vi "FPGAcode.vi"() -> ()   [LabVIEW 2013]
uses:
  <vilib>/Platform/TimedLoop/XDataNode/timing_clust.ctl
  <vilib>/Platform/TimedLoop/XDataNode/nitl_modes.ctl
  <vilib>/Platform/TimedLoop/XDataNode/wakeup.ctl
  <vilib>/rvi/Emulation/niFpgaSctlEmulationGetInTimedLoop.vi
  <vilib>/rvi/Emulation/niFpgaEmulationReportErrorSimple.vi
  <vilib>/rvi/Emulation/niFpgaGetClockAttributes.vi
  <vilib>/rvi/Emulation/niFpgaCriticalErrorInLSC.vi
  <vilib>/rvi/eio/common/nirviEmuTemplateMethod_errors.vi
  <vilib>/Platform/TimedLoop/XDataNode/XDataNode.xnode
  <vilib>/eio/EIONode/EIONode.xnode
  <vilib>/Platform/TimedLoop/XDataNode/XDNodeRunTimeDep.lvlib
panel:
  out "Del Not Armed?":bool
  out "Not Armed?":bool
  in  "Reset One Shot":bool
  in  "One Shot":bool
  out "Filter 1 Detector 3 Correlation":i32
  in  "Filter 2 threshold":i32=1000
  out "Filter 2 Detector 3 Correlation":i32
  in  "Filter 1 threshold":i32=1000
  in  "Filter 3 threshold":i32=1000
  out "Filter 3 Detector 3 Correlation":i32
  in  "Filter 4 threshold":i32=1000
  out "Filter 4 Detector 3 Correlation":i32
  in  "Filter 5 threshold":i32
  out "Filter 5 Detector 3 Correlation":i32
  in  "Filter 6 threshold":i32
  out "Filter 6 Detector 3 Correlation":i32
  in  "Filter 7 threshold":i32
  out "Filter 7 Detector 3 Correlation":i32
  out "Plates":bool
  in  "High Charge Limit":i16
  in  "Low Charge Limit":i16
  in  "High Velocity Count":i32
  in  "Low Velocity Count":i32
  in  "High Mass Limit":i64
  in  "Low Mass Limit":i64
  in  "Mult1":fxp<+,16,7>
  out "Delay1":bool
  out "IO Module\\AI 0":i16
  out "IO Module\\AI 1":i16
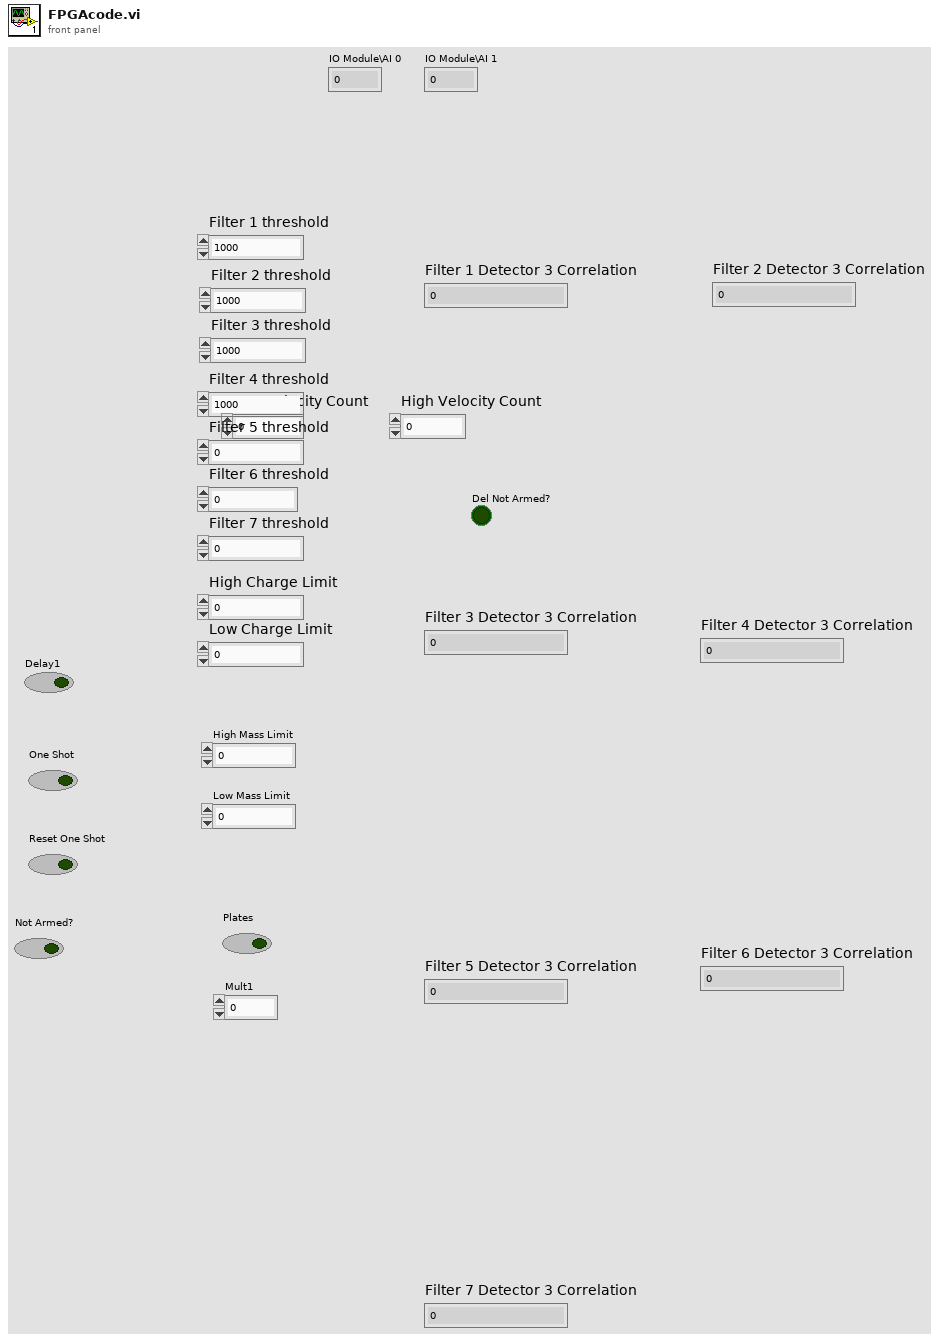
[diagram p1: front panel]
types:
  T1 = typedef "XDNodeRunTimeDep.lvlib/timing_clust.ctl" = cluster{"Expected End [f-1]":u64, "Actual End [f-1]":u64, "Finished Late? [f-1]":bool, "Expected End [i-1]":u64, "Actual End [i-1]":u64, "Finished Late? [i-1]":bool, "Expected Start [i]":u64, "Actual Start [i]":u64, "Expected Start [f]":u64, "Actual Start [f]":u64, "Source Name":string, "Structure Name":string, "Period":i64, "Deadline":i64, "Offset":i64, "Start":i64, "Priority":i32, "Timeout":i32, "Mode":T2, "Wakeup Reason":T3, "Error":errorcluster, "Source Type":string, "Secondary Source Type":string, "Global End Time":u64, "Global Start Time":u64, "Frame Duration":u64, "Iteration Duration":u64, "Assigned CPU":i32, "I/O Scan Engine Mode":u32}
  T2 = typedef "XDNodeRunTimeDep.lvlib/nitl_modes.ctl" = enum32{"No Change", "Process missed periods, maintain original phase", "Discard missed periods, maintain original phase", "Process missed periods, ignore original phase", "Discard missed periods, ignore original phase"}
  T3 = typedef "XDNodeRunTimeDep.lvlib/wakeup.ctl" = enum32{"Normal", "Aborted", "Asynchronous wakeup", "Timing source error", "Timed loop error", "Timeout"}
  T4 = cluster{"Separation cut off 1":i32, "Filter Number":i32, "Separation cut off 2":i32}
  T5 = cluster{"Old Average":i32, "New Average":i32, "Current State":u8, "Detector 1 Correlation":i32, "Detector 3 Correlation":i32, "Velocity Count":i32, "Detector Counter in":i32, "Timeout Count in":i32, "Measured Charge in":i32, "Filter Threshold":i32, "High Correlation in":i32, "Offset":i32, "Offset Average":i32, "Measured Velocity In":i32, "Mult Cluster":cluster{"Mult1":fxp<+,16,7>, "Mult1 Use?":bool}, "Final Delay Count In":u16, "Delay1 In":i32}
  T6 = cluster{"High Charge Limit":i16, "Low Charge Limit":i16, "Low Velocity Count":i32, "High Velocity Count":i32, "Low Velocity Count":i32, fxp<+,30,25>, "High Mass Limit":i64, "Low Mass Limit":i64}
  T7 = cluster{"Average Out":i32, "Next State":u8, "Velocity Count out":i32, "Detector counter out":i32, "Timeout count out":u32, "Measured Charge Out":i32, "High Correlation Out":i32, "Plates":bool, "Offset Out":i32, "Measured Velocity Out":i32, "Final Delay Count Out":u16, "Out1":bool, "Delay1":i32}
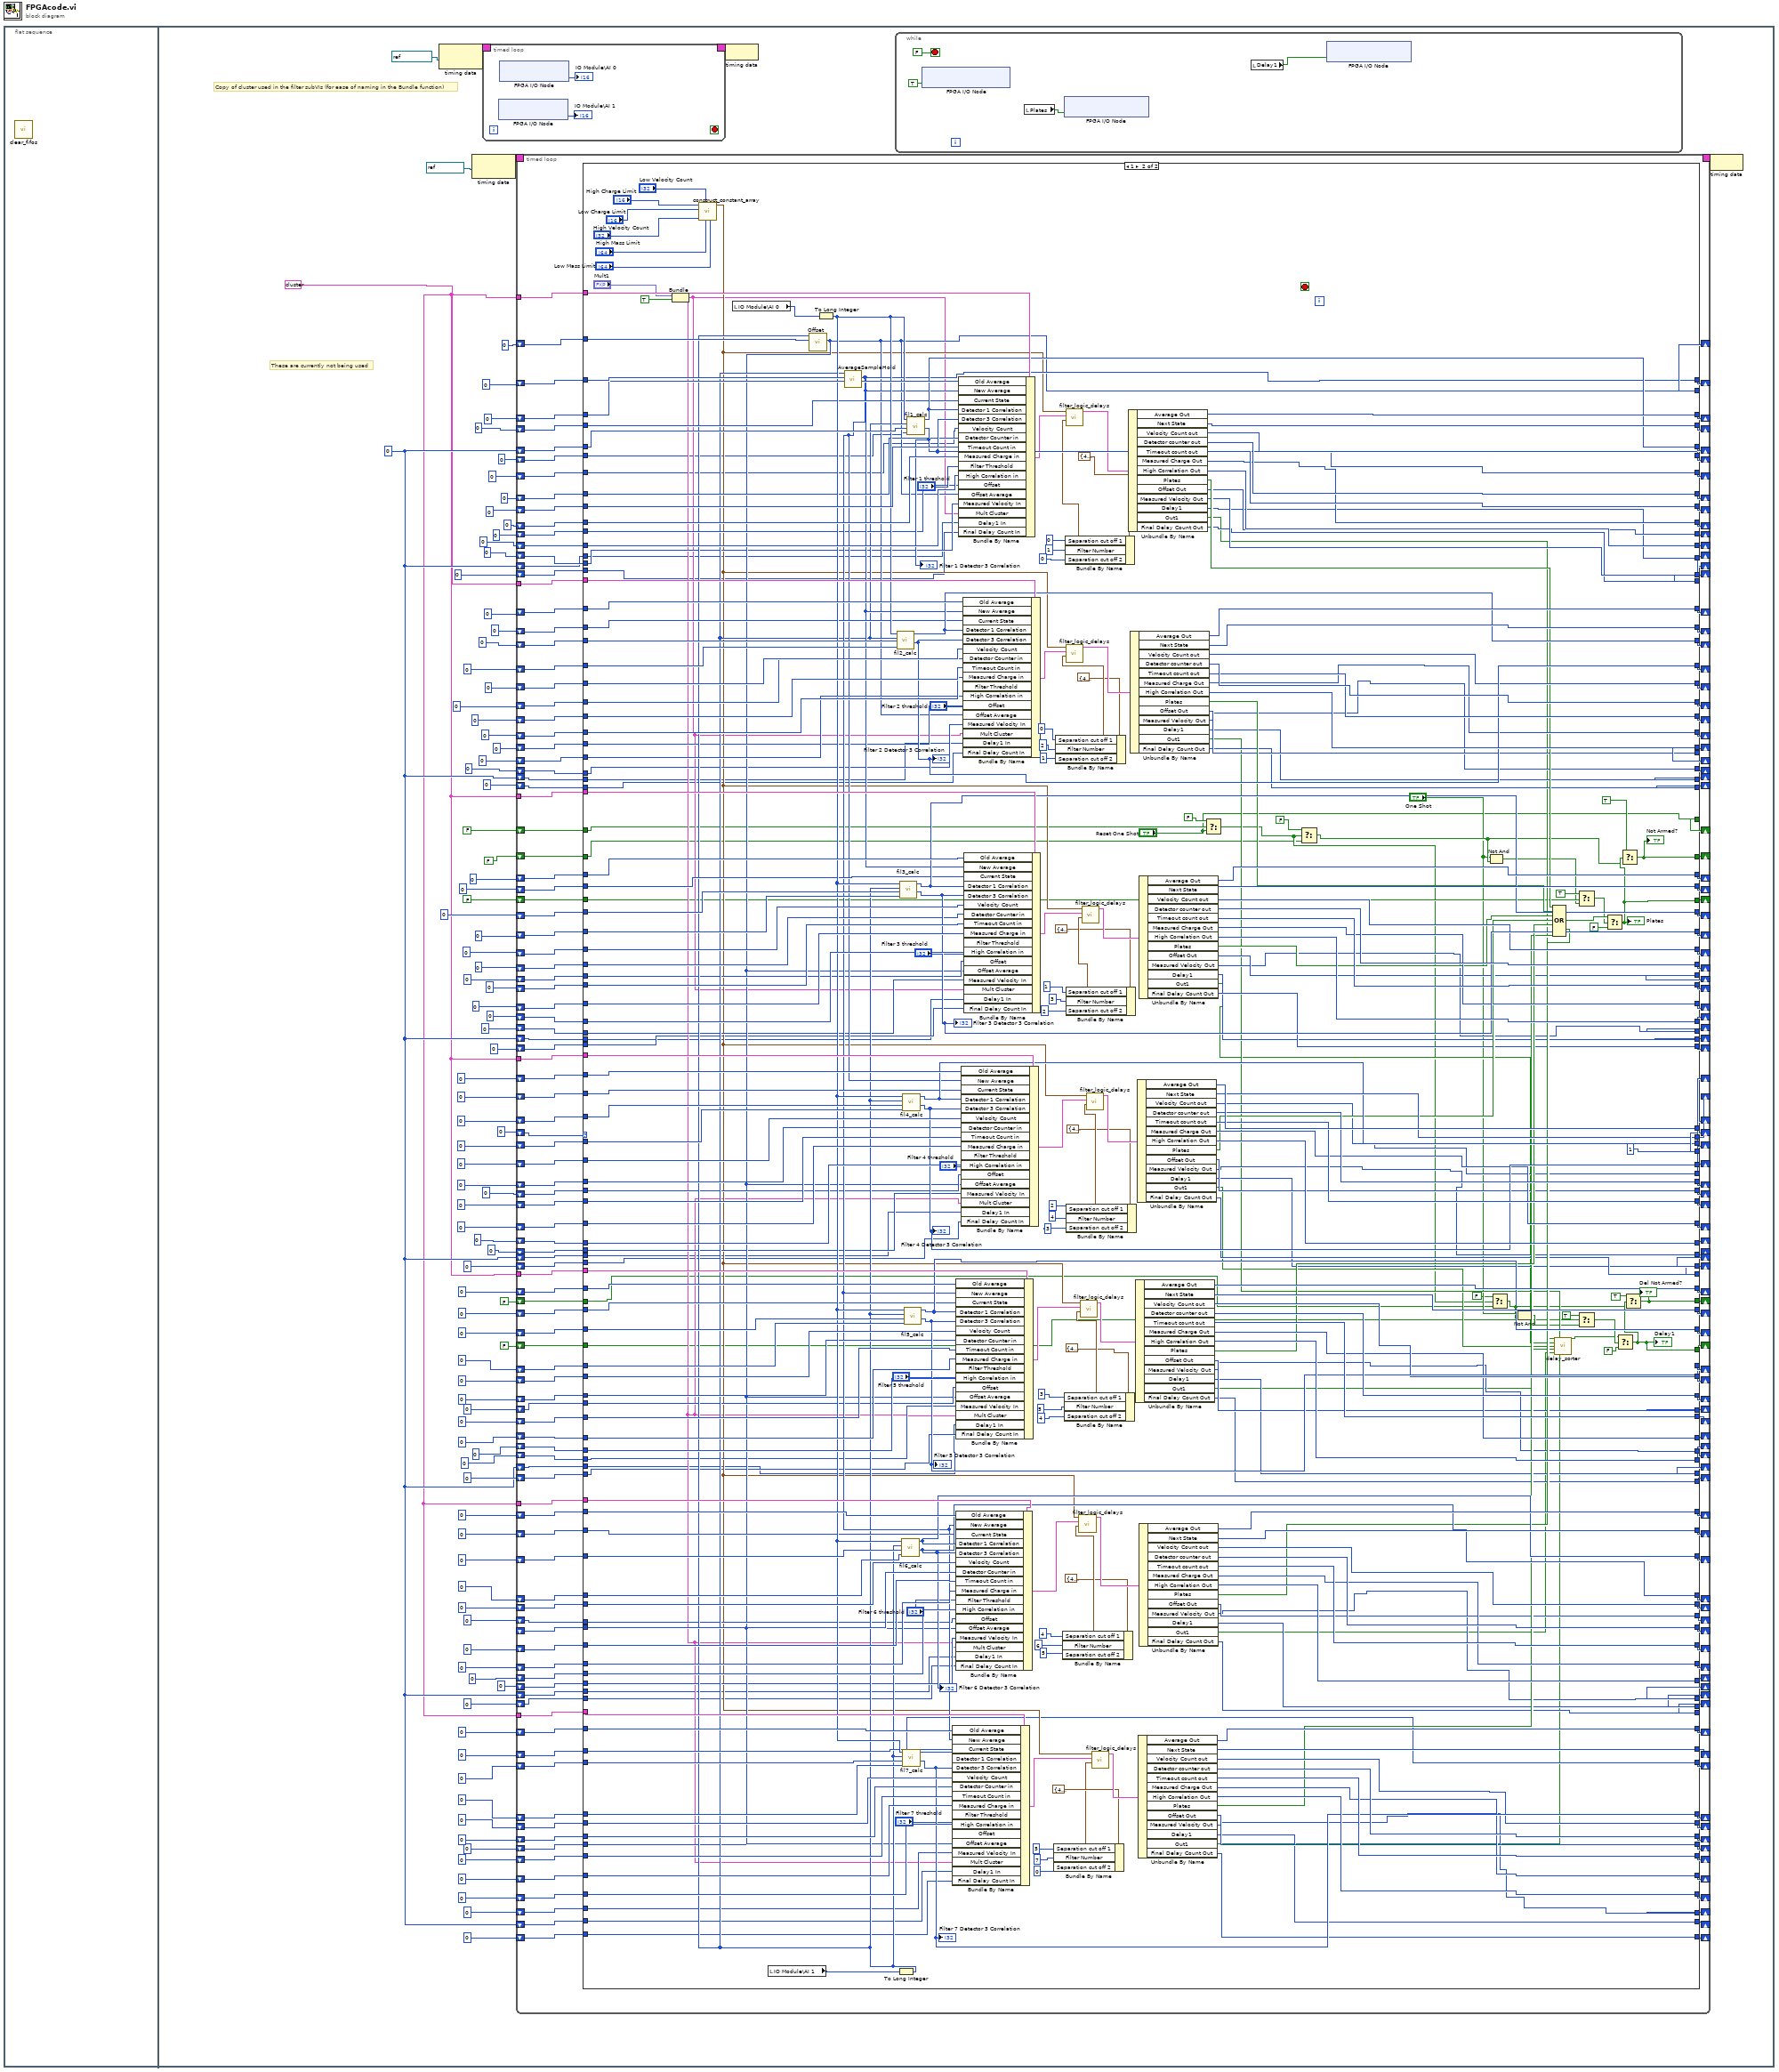
[diagram p0: block diagram]
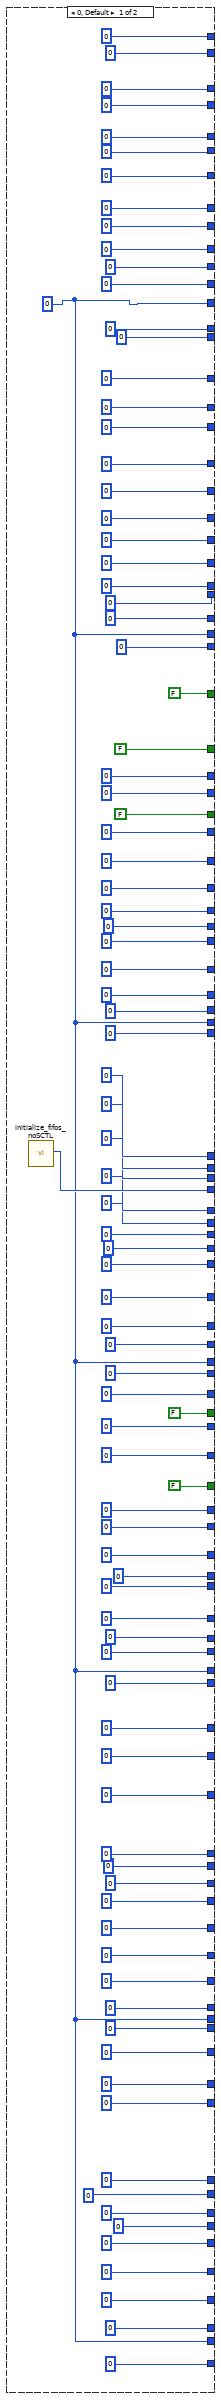
[diagram p2: hidden frame]
diagram:
  n1 = flat-sequence {
    frame #0 {
      n2 = call "clear_fifos.vi"() -> ()  [unwired: 1 in]
    }
    frame #1 {
      w4 = T5 {"Old Average"=0, "New Average"=0, "Current State"=0, "Detector 1 Correlation"=0, "Detector 3 Correlation"=0, "Velocity Count"=0, "Detector Counter in"=0, "Timeout Count in"=0, "Measured Charge in"=0, "Filter Threshold"=0, "High Correlation in"=0, "Offset"=0, "Offset Average"=0, "Measured Velocity In"=0, "Mult Cluster"={"Mult1"=0.0, "Mult1 Use?"=FALSE}, "Final Delay Count In"=0, "Delay1 In"=0} ("Variables Cluster")
      w7 = 0 ("Detector 1 Correlation Out")
      # "These are currently not being used"
      # "Copy of cluster used in the filter subVIs (for ease of naming in the Bundle function)"
      n3 = node-c288(refnum<k21> "AI Clock" ("Source Name")) -> (w34:T1)
      n4 = node-c288(refnum<k21> "26 MHz" ("Source Name")) -> (w98:T1)
      n5 = timed-loop {
        timing: w34 -> [_]
        timing-out: [_] -> w33
        stop <- _ stop-if-true
        n6 = xnode "FPGA I/O Node"() -> ("IO Module\\AI 1"=→"IO Module\\AI 1":i16)  [unwired: 1 in, 1 out]
        n7 = xnode "FPGA I/O Node"() -> ("IO Module\\AI 0"=→"IO Module\\AI 0":i16)  [unwired: 1 in, 1 out]
      }
      n8 = timed-loop {
        timing: w98 -> [_]
        timing-out: [_] -> w97
        shift-right: [w308] -> _
        shift-left: 0 ("Velocity Count out") -> [w230]
        shift-right: [w309] -> _
        shift-left: 0 ("Detector 1 Correlation out") -> [w231]
        shift-right: [w195] -> _
        shift-left: 0 ("Detector counter out") -> [w232]
        shift-right: [w226] -> _
        shift-left: 0 ("Next State") -> [w233]
        shift-right: [w194] -> _
        shift-left: 0 ("Detector 3 Correlation out") -> [w229]
        shift-right: [w307] -> _
        shift-left: 0 ("Timeout count out") -> [w228]
        shift-right: [w222] -> _
        shift-left: 0 ("Next State") -> [w225]
        shift-right: [w221] -> _
        shift-left: 0 ("Detector counter out") -> [w224]
        shift-right: [w193] -> _
        shift-left: 0 ("Detector 1 Correlation out") -> [w301]
        shift-right: [w298] -> _
        shift-left: 0 ("Velocity Count out") -> [w300]
        shift-right: [w297] -> _
        shift-left: u32 0 ("Detector 3 Correlation out") -> [w299]
        shift-right: [w292] -> _
        shift-left: 0 ("Timeout count out") -> [w293]
        shift-right: [w216] -> _
        shift-left: 0 ("Next State") -> [w219]
        shift-right: [w191] -> _
        shift-left: 0 ("Detector counter out") -> [w289]
        shift-right: [w287] -> _
        shift-left: 0 ("Detector 1 Correlation out") -> [w288]
        shift-right: [w285] -> _
        shift-left: u32 0 ("Velocity Count out") -> [w286]
        shift-right: [w190] -> _
        shift-left: 0 ("Detector 3 Correlation out") -> [w284]
        shift-right: [w283] -> _
        shift-left: 0 ("Timeout count out") -> [w218]
        shift-right: [w310] -> _
        shift-left: u8 0 ("High Correlation Out") -> [w313]
        shift-right: [w302] -> _
        shift-left: u8 0 ("High Correlation Out") -> [w303]
        shift-right: [w217] -> _
        shift-left: 0 ("High Correlation Out") -> [w220]
        shift-right: [w311] -> _
        shift-left: 0 ("Measured Charge Out") -> [w314]
        shift-right: [w304] -> _
        shift-left: 0 ("Measured Charge Out") -> [w305]
        shift-right: [w291] -> _
        shift-left: u8 0 ("Measured Charge Out") -> [w290]
        shift-right: [w181] -> _
        shift-left: 0 ("Output New Average") -> [w315]
        shift-right: [w227] -> _
        shift-left: w7 -> [w234]
        tunnel: w4 -> [w312]
        shift-right: [w192] -> _
        shift-left: 0 ("High Sample Out") -> [w295]
        shift-right: [w296] -> _
        shift-left: 0 ("High Correlation Out") -> [w223]
        tunnel: w4 -> [w306]
        tunnel: w4 -> [w294]
        shift-right: [w282] -> _
        shift-left: 0 ("Average Out") -> [w281]
        shift-right: [w280] -> _
        shift-left: u8 0 ("Next State") -> [w279]
        shift-right: [w212] -> _
        shift-left: 0 ("Detector 1 Correlation out") -> [w214]
        shift-right: [w211] -> _
        shift-left: 0 ("Detector 3 Correlation out") -> [w213]
        shift-right: [w189] -> _
        shift-left: 0 ("Velocity Count out") -> [w278]
        shift-right: [w277] -> _
        shift-left: 0 ("Detector counter out") -> [w276]
        shift-right: [w275] -> _
        shift-left: u32 0 ("Timeout count out") -> [w274]
        shift-right: [w188] -> _
        shift-left: 0 ("Measured Charge Out") -> [w273]
        shift-right: [w272] -> _
        shift-left: 0 ("High Correlation Out") -> [w215]
        tunnel: w4 -> [w271]
        shift-right: [w269] -> _
        shift-left: 0 ("Average Out") -> [w268]
        shift-right: [w267] -> _
        shift-left: u8 0 ("Next State") -> [w266]
        shift-right: [w207] -> _
        shift-left: 0 ("Detector 1 Correlation out") -> [w210]
        shift-right: [w206] -> _
        shift-left: 0 ("Detector 3 Correlation out") -> [w209]
        shift-right: [w187] -> _
        shift-left: 0 ("Velocity Count out") -> [w265]
        shift-right: [w264] -> _
        shift-left: 0 ("Detector counter out") -> [w263]
        shift-right: [w262] -> _
        shift-left: u32 0 ("Timeout count out") -> [w261]
        shift-right: [w186] -> _
        shift-left: 0 ("Measured Charge Out") -> [w260]
        shift-right: [w259] -> _
        shift-left: 0 ("High Correlation Out") -> [w208]
        tunnel: w4 -> [w270]
        shift-right: [w257] -> _
        shift-left: 0 ("Average Out") -> [w255]
        shift-right: [w256] -> _
        shift-left: u8 0 ("Next State") -> [w252]
        shift-right: [w202] -> _
        shift-left: 0 ("Detector 1 Correlation out") -> [w205]
        shift-right: [w201] -> _
        shift-left: 0 ("Detector 3 Correlation out") -> [w204]
        shift-right: [w184] -> _
        shift-left: 0 ("Velocity Count out") -> [w254]
        shift-right: [w251] -> _
        shift-left: _ -> [w253]
        shift-right: [w250] -> _
        shift-left: u32 0 ("Timeout count out") -> [w249]
        shift-right: [w185] -> _
        shift-left: 0 ("Measured Charge Out") -> [w248]
        shift-right: [w247] -> _
        shift-left: 0 ("High Correlation Out") -> [w203]
        tunnel: w4 -> [w258]
        shift-right: [w245] -> _
        shift-left: 0 ("Average Out") -> [w244]
        shift-right: [w243] -> _
        shift-left: u8 0 ("Next State") -> [w235]
        shift-right: [w197] -> _
        shift-left: 0 ("Detector 1 Correlation out") -> [w200]
        shift-right: [w196] -> _
        shift-left: 0 ("Detector 3 Correlation out") -> [w199]
        shift-right: [w183] -> _
        shift-left: 0 ("Velocity Count out") -> [w242]
        shift-right: [w241] -> _
        shift-left: 0 ("Detector counter out") -> [w240]
        shift-right: [w239] -> _
        shift-left: u32 0 ("Timeout count out") -> [w238]
        shift-right: [w182] -> _
        shift-left: 0 ("Measured Charge Out") -> [w237]
        shift-right: [w236] -> _
        shift-left: 0 ("High Correlation Out") -> [w198]
        tunnel: w4 -> [w246]
        shift-right: [w179] -> _
        shift-left: i16 0 -> [w180]
        shift-right: [w177] -> _
        shift-left: 0 -> [w178]
        shift-right: [w176] -> _
        shift-left: 0 -> [w173]
        shift-right: [w174] -> _
        shift-left: 0 -> [w175]
        shift-right: [w171] -> _
        shift-left: 0 ("Offset Out") -> [w172]
        shift-right: [w170] -> _
        shift-left: 0 ("Offset Out") -> [w169]
        shift-right: [w168] -> _
        shift-left: 0 ("Offset Out") -> [w167]
        shift-right: [w166] -> _
        shift-left: 0 ("Offset Out") -> [w165]
        shift-right: [w164] -> _
        shift-left: 0 ("Offset Out") -> [w163]
        shift-right: [w161] -> _
        shift-left: 0 -> [w162]
        shift-right: [w160] -> _
        shift-left: 0 -> [w149]
        shift-right: [w159] -> _
        shift-left: 0 -> [w150]
        shift-right: [w158] -> _
        shift-left: 0 -> [w151]
        shift-right: [w157] -> _
        shift-left: 0 -> [w152]
        shift-right: [w156] -> _
        shift-left: 0 -> [w153]
        shift-right: [w155] -> _
        shift-left: 0 ("Measured Velocity Out") -> [w154]
        shift-right: [w148] -> _
        shift-left: w7 -> [w146]
        shift-right: [w147] -> _
        shift-left: u32 0 ("Final Delay Count Out") -> [w145]
        shift-right: [w144] -> _
        shift-left: w7 -> [w142]
        shift-right: [w143] -> _
        shift-left: u32 0 ("Final Delay Count Out") -> [w141]
        shift-right: [w140] -> _
        shift-left: w7 -> [w138]
        shift-right: [w139] -> _
        shift-left: u32 0 ("Final Delay Count Out") -> [w137]
        shift-right: [w136] -> _
        shift-left: w7 -> [w134]
        shift-right: [w135] -> _
        shift-left: u32 0 ("Final Delay Count Out") -> [w133]
        shift-right: [w132] -> _
        shift-left: w7 -> [w130]
        shift-right: [w131] -> _
        shift-left: u32 0 ("Final Delay Count Out") -> [w129]
        shift-right: [w128] -> _
        shift-left: w7 -> [w126]
        shift-right: [w127] -> _
        shift-left: u32 0 ("Final Delay Count Out") -> [w125]
        shift-right: [w124] -> _
        shift-left: w7 -> [w122]
        shift-right: [w123] -> _
        shift-left: u32 0 ("Final Delay Count Out") -> [w121]
        shift-right: [w119] -> _
        shift-left: FALSE -> [w120]
        shift-right: [w118] -> _
        shift-left: FALSE ("f") -> [w117]
        shift-right: [w116] -> _
        shift-left: FALSE ("Reset One Shot") -> [w115]
        shift-right: [w111] -> _
        shift-left: FALSE -> [w114]
        shift-right: [w112] -> _
        shift-left: FALSE -> [w113]
        stop <- _ stop-if-true
        n9 = case shown="1" w180 {
          tunnel: w315 -> [_ w715]
          tunnel: w314 -> [_ w714]
          tunnel: w313 -> [_ w549]
          tunnel: w312 -> [_ w713]
          tunnel: [0 ("Average Out") w712] -> w311
          tunnel: [u16 0 ("Next State") w711] -> w310
          tunnel: [0 ("Detector counter out") w710] -> w309
          tunnel: [u32 0 ("Timeout count out") w709] -> w308
          tunnel: [0 ("High Correlation Out") w708] -> w307
          tunnel: w306 -> [_ w707]
          tunnel: w305 -> [_ w706]
          tunnel: [0 ("Average Out") w705] -> w304
          tunnel: w303 -> [_ w548]
          tunnel: [u16 0 ("Next State") w704] -> w302
          tunnel: w301 -> [_ w703]
          tunnel: w300 -> [_ w541]
          tunnel: w299 -> [_ w702]
          tunnel: [0 ("Detector counter out") w701] -> w298
          tunnel: [u32 0 ("Timeout count out") w700] -> w297
          tunnel: [0 ("High Correlation Out") w699] -> w296
          tunnel: w295 -> [_ w698]
          tunnel: w294 -> [_ w697]
          tunnel: w293 -> [_ w696]
          tunnel: [0 ("Average Out") w695] -> w292
          tunnel: [u16 0 ("Next State") w694] -> w291
          tunnel: w290 -> [_ w547]
          tunnel: w289 -> [_ w693]
          tunnel: w288 -> [_ w540]
          tunnel: [0 ("Detector counter out") w692] -> w287
          tunnel: w286 -> [_ w691]
          tunnel: [u32 0 ("Timeout count out") w690] -> w285
          tunnel: w284 -> [_ w689]
          tunnel: [0 ("High Correlation Out") w688] -> w283
          tunnel: [0 ("Average Out") w687] -> w282
          tunnel: w281 -> [_ w686]
          tunnel: [u16 0 ("Next State") w685] -> w280
          tunnel: w279 -> [_ w546]
          tunnel: w278 -> [_ w684]
          tunnel: [0 ("Detector counter out") w683] -> w277
          tunnel: w276 -> [_ w539]
          tunnel: [u32 0 ("Timeout count out") w682] -> w275
          tunnel: w274 -> [_ w681]
          tunnel: w273 -> [_ w680]
          tunnel: [0 ("High Correlation Out") w679] -> w272
          tunnel: w271 -> [_ w678]
          tunnel: w270 -> [_ w677]
          tunnel: [0 ("Average Out") w676] -> w269
          tunnel: w268 -> [_ w675]
          tunnel: [u16 0 ("Next State") w674] -> w267
          tunnel: w266 -> [_ w545]
          tunnel: w265 -> [_ w673]
          tunnel: [0 ("Detector counter out") w672] -> w264
          tunnel: w263 -> [_ w538]
          tunnel: [u32 0 ("Timeout count out") w671] -> w262
          tunnel: w261 -> [_ w670]
          tunnel: w260 -> [_ w669]
          tunnel: [0 ("High Correlation Out") w668] -> w259
          tunnel: w258 -> [_ w667]
          tunnel: [0 ("Average Out") w666] -> w257
          tunnel: [u16 0 ("Next State") w665] -> w256
          tunnel: w255 -> [_ w664]
          tunnel: w254 -> [_ w663]
          tunnel: w253 -> [_ w537]
          tunnel: w252 -> [_ w544]
          tunnel: [0 ("Detector counter out") w662] -> w251
          tunnel: [u32 0 ("Timeout count out") w661] -> w250
          tunnel: w249 -> [_ w660]
          tunnel: w248 -> [_ w659]
          tunnel: [0 ("High Correlation Out") w658] -> w247
          tunnel: w246 -> [_ w657]
          tunnel: [0 ("Average Out") w656] -> w245
          tunnel: w244 -> [_ w655]
          tunnel: [u16 0 ("Next State") w654] -> w243
          tunnel: w242 -> [_ w653]
          tunnel: [0 ("Detector counter out") w652] -> w241
          tunnel: w240 -> [_ w536]
          tunnel: [u32 0 ("Timeout count out") w651] -> w239
          tunnel: w238 -> [_ w650]
          tunnel: w237 -> [_ w649]
          tunnel: [0 ("High Correlation Out") w648] -> w236
          tunnel: w235 -> [_ w543]
          tunnel: w234 -> [_ w647]
          tunnel: w233 -> [_ w444]
          tunnel: w232 -> [_ w445]
          tunnel: w231 -> [_ w542]
          tunnel: w230 -> [_ w646]
          tunnel: w229 -> [_ w645]
          tunnel: w228 -> [_ w644]
          tunnel: [0 ("Detector 1 Correlation Out") w643] -> w227
          tunnel: [0 ("Detector 3 Correlation Out") w642] -> w226
          tunnel: w225 -> [_ w641]
          tunnel: w224 -> [_ w640]
          tunnel: w223 -> [_ w639]
          tunnel: [0 ("Detector 1 Correlation Out") w638] -> w222
          tunnel: [0 ("Detector 3 Correlation Out") w637] -> w221
          tunnel: w220 -> [_ w636]
          tunnel: w219 -> [_ w635]
          tunnel: w218 -> [_ w634]
          tunnel: [0 ("Detector 1 Correlation Out") w633] -> w217
          tunnel: [0 ("Detector 3 Correlation Out") w632] -> w216
          tunnel: w215 -> [_ w631]
          tunnel: w214 -> [_ w630]
          tunnel: w213 -> [_ w629]
          tunnel: [0 ("Detector 1 Correlation Out") w628] -> w212
          tunnel: [0 ("Detector 3 Correlation Out") w627] -> w211
          tunnel: w210 -> [_ w626]
          tunnel: w209 -> [_ w625]
          tunnel: w208 -> [_ w624]
          tunnel: [0 ("Detector 1 Correlation Out") w623] -> w207
          tunnel: [0 ("Detector 3 Correlation Out") w622] -> w206
          tunnel: w205 -> [_ w621]
          tunnel: w204 -> [_ w620]
          tunnel: w203 -> [_ w619]
          tunnel: [0 ("Detector 1 Correlation Out") w618] -> w202
          tunnel: [0 ("Detector 3 Correlation Out") w617] -> w201
          tunnel: w200 -> [_ w616]
          tunnel: w199 -> [_ w615]
          tunnel: w198 -> [_ w614]
          tunnel: [0 ("Detector 1 Correlation Out") w479] -> w197
          tunnel: [0 ("Detector 3 Correlation Out") w613] -> w196
          tunnel: [0 ("Velocity Count out") w612] -> w195
          tunnel: [0 ("Measured Charge Out") w611] -> w194
          tunnel: [0 ("Velocity Count out") w610] -> w193
          tunnel: [0 ("Measured Charge Out") w609] -> w192
          tunnel: [0 ("Velocity Count out") w608] -> w191
          tunnel: [0 ("Measured Charge Out") w607] -> w190
          tunnel: [0 ("Velocity Count out") w535] -> w189
          tunnel: [0 ("Measured Charge Out") w606] -> w188
          tunnel: [0 ("Velocity Count out") w605] -> w187
          tunnel: [0 ("Measured Charge Out") w604] -> w186
          tunnel: [0 ("Measured Charge Out") w603] -> w185
          tunnel: [0 ("Velocity Count out") w602] -> w184
          tunnel: [0 ("Velocity Count out") w601] -> w183
          tunnel: [0 ("Measured Charge Out") w600] -> w182
          tunnel: [0 ("Output New Average") w534] -> w181
          tunnel: [w408 i16 1 ("Output State")] -> w179
          tunnel: w178 -> [_ w531]
          tunnel: [0 ("Offset Out") w530] -> w177
          tunnel: [0 ("Offset Out") w529] -> w176
          tunnel: w175 -> [_ w528]
          tunnel: [0 ("Output New Average") w517] -> w174
          tunnel: w173 -> [_ w526]
          tunnel: w172 -> [_ w525]
          tunnel: [0 ("Offset Out") w524] -> w171
          tunnel: [0 ("Offset Out") w523] -> w170
          tunnel: w169 -> [_ w522]
          tunnel: [0 ("Offset Out") w521] -> w168
          tunnel: w167 -> [_ w520]
          tunnel: [0 ("Offset Out") w519] -> w166
          tunnel: w165 -> [_ w518]
          tunnel: [0 ("Offset Out") w516] -> w164
          tunnel: w163 -> [_ w515]
          tunnel: w162 -> [_ w510]
          tunnel: [0 ("Measured Velocity Out") w503] -> w161
          tunnel: [0 ("Measured Velocity Out") w502] -> w160
          tunnel: [0 ("Measured Velocity Out") w501] -> w159
          tunnel: [0 ("Measured Velocity Out") w500] -> w158
          tunnel: [0 ("Measured Velocity Out") w499] -> w157
          tunnel: [0 ("Measured Velocity Out") w498] -> w156
          tunnel: [0 ("Measured Velocity Out") w497] -> w155
          tunnel: w154 -> [_ w509]
          tunnel: w153 -> [_ w508]
          tunnel: w152 -> [_ w507]
          tunnel: w151 -> [_ w506]
          tunnel: w150 -> [_ w505]
          tunnel: w149 -> [_ w504]
          tunnel: [w321 w474] -> w148
          tunnel: [u32 0 ("Final Delay Count Out") w492] -> w147
          tunnel: w146 -> [_ w491]
          tunnel: w145 -> [_ w490]
          tunnel: [w321 w489] -> w144
          tunnel: [u32 0 ("Final Delay Count Out") w488] -> w143
          tunnel: w142 -> [_ w487]
          tunnel: w141 -> [_ w486]
          tunnel: [w321 w473] -> w140
          tunnel: [u32 0 ("Final Delay Count Out") w485] -> w139
          tunnel: w138 -> [_ w466]
          tunnel: w137 -> [_ w484]
          tunnel: [w321 w472] -> w136
          tunnel: [u32 0 ("Final Delay Count Out") w483] -> w135
          tunnel: w134 -> [_ w465]
          tunnel: w133 -> [_ w482]
          tunnel: [w321 w471] -> w132
          tunnel: [u32 0 ("Final Delay Count Out") w481] -> w131
          tunnel: w130 -> [_ w464]
          tunnel: w129 -> [_ w480]
          tunnel: [w321 w470] -> w128
          tunnel: [u32 0 ("Final Delay Count Out") w478] -> w127
          tunnel: w126 -> [_ w463]
          tunnel: w125 -> [_ w477]
          tunnel: [w321 w469] -> w124
          tunnel: [u32 0 ("Final Delay Count Out") w476] -> w123
          tunnel: w122 -> [_ w462]
          tunnel: w121 -> [_ w475]
          tunnel: w120 -> [_ w410]
          tunnel: [FALSE ("t") w430] -> w119
          tunnel: [FALSE ("f") w442] -> w118
          tunnel: w117 -> [_ w441]
          tunnel: [FALSE ("Reset One Shot") "Reset One Shot"] -> w116
          tunnel: w115 -> [_ w428]
          tunnel: w114 -> [_ w411]
          tunnel: w113 -> [_ w417]
          tunnel: [FALSE ("Delay1") w416] -> w112
          tunnel: [FALSE w413] -> w111
          frame 0, Default {
            w321 = 0
            n10 = call "initialize_fifos_noSCTL.vi"() -> ("Output State"=w408:i16)  [unwired: 11 in]
          }
          frame 1 {
            n11 = Bundle("Mult1"="Mult1", TRUE) -> (w493:cluster{"Mult1":fxp<+,16,7>, bool})  [unwired: 1 in]
            n12 = call "construct_constant_array.vi"("Low Mass Limit"="Low Mass Limit", "High Mass Limit"="High Mass Limit", "Low Velocity Count"="Low Velocity Count", "High Velocity Count"="High Velocity Count", "Low Charge Limit"="Low Charge Limit", "High Charge Limit"="High Charge Limit") -> ("constants cluster"=w494:T6)  [unwired: 5 in]
            n13 = local read "IO Module\\AI 0"() -> (w533:i16)
            n14 = local read "IO Module\\AI 1"() -> (w532:i16)
            n15 = To Long Integer(number=w533) -> (32bit integer=w558:i32)
            n16 = To Long Integer(number=w532) -> (32bit integer=w527:i32)
            n17 = call "Offset.vi"("Previous Average"=w528, "Input Value"=w527) -> ("Output New Average"=w517:i32)  [unwired: 7 in]
            n18 = call "AverageSampleHold.vi"("Previous Average"=w715, "Input Value"=w527) -> ("Output New Average"=w534:i32)  [unwired: 7 in]
            n19 = call "fil2_calc.vi"("Detector 3 Correlation In"=w640, "Detector 1 Correlation In"=w641, "AI1"=w527, "AI0"=w558) -> ("Detector 3 Correlation Out"=w637:i32, "Detector 1 Correlation Out"=w638:i32)  [unwired: 4 in]
            "Filter 2 Detector 3 Correlation" <- w637
            n20 = call "fil3_calc.vi"("Detector 3 Correlation In"=w635, "Detector 1 Correlation In"=w636, "AI1"=w527, "AI0"=w558) -> ("Detector 3 Correlation Out"=w632:i32, "Detector 1 Correlation Out"=w633:i32)  [unwired: 4 in]
            "Filter 3 Detector 3 Correlation" <- w632
            n21 = call "fil6_calc.vi"("Detector 3 Correlation In"=w620, "Detector 1 Correlation In"=w621, "AI1"=w527, "AI0"=w558) -> ("Detector 3 Correlation Out"=w617:i32, "Detector 1 Correlation Out"=w618:i32)  [unwired: 4 in]
            "Filter 6 Detector 3 Correlation" <- w617
            n22 = call "fil4_calc.vi"("Detector 3 Correlation In"=w629, "Detector 1 Correlation In"=w630, "AI1"=w527, "AI0"=w558) -> ("Detector 3 Correlation Out"=w627:i32, "Detector 1 Correlation Out"=w628:i32)  [unwired: 4 in]
            "Filter 4 Detector 3 Correlation" <- w627
            n23 = call "fil7_calc.vi"("Detector 3 Correlation In"=w615, "Detector 1 Correlation In"=w616, "AI1"=w527, "AI0"=w558) -> ("Detector 3 Correlation Out"=w613:i32, "Detector 1 Correlation Out"=w479:i32)  [unwired: 4 in]
            "Filter 7 Detector 3 Correlation" <- w613
            n24 = call "fil5_calc.vi"("Detector 3 Correlation In"=w625, "Detector 1 Correlation In"=w626, "AI1"=w527, "AI0"=w558) -> ("Detector 3 Correlation Out"=w622:i32, "Detector 1 Correlation Out"=w623:i32)  [unwired: 4 in]
            "Filter 5 Detector 3 Correlation" <- w622
            n25 = call "fil1_calc.vi"("Detector 3 Correlation In"=w444, "Detector 1 Correlation In"=w647, "AI1"=w527, "AI0"=w558) -> ("Detector 3 Correlation Out"=w642:i32, "Detector 1 Correlation Out"=w643:i32)  [unwired: 4 in]
            "Filter 1 Detector 3 Correlation" <- w642
            n26 = Bundle By Name(cluster=w657, "Old Average"=w655, "New Average"=w534, "Current State"=w543, "Detector 1 Correlation"=w479, "Detector 3 Correlation"=w613, "Velocity Count"=w653, "Detector Counter in"=w536, "Timeout Count in"=w650, "Measured Charge in"=w649, "Filter Threshold"="Filter 7 threshold", "High Correlation in"=w614, "Offset"=w515, "Offset Average"=w517, "Measured Velocity In"=w509, "Mult Cluster"=w493, "Delay1 In"=w462, "Final Delay Count In"=w475) -> (w432:T5)
            n27 = Bundle By Name(cluster=w667, "Old Average"=w664, "New Average"=w534, "Current State"=w544, "Detector 1 Correlation"=w618, "Detector 3 Correlation"=w617, "Velocity Count"=w663, "Detector Counter in"=w537, "Timeout Count in"=w660, "Measured Charge in"=w659, "Filter Threshold"="Filter 6 threshold", "High Correlation in"=w619, "Offset"=w518, "Offset Average"=w517, "Measured Velocity In"=w508, "Mult Cluster"=w493, "Delay1 In"=w463, "Final Delay Count In"=w477) -> (w433:T5)
            n28 = Bundle By Name(cluster=w677, "Old Average"=w675, "New Average"=w534, "Current State"=w545, "Detector 1 Correlation"=w623, "Detector 3 Correlation"=w622, "Velocity Count"=w673, "Detector Counter in"=w538, "Timeout Count in"=w670, "Measured Charge in"=w669, "Filter Threshold"="Filter 5 threshold", "High Correlation in"=w624, "Offset"=w520, "Offset Average"=w517, "Measured Velocity In"=w507, "Mult Cluster"=w493, "Delay1 In"=w464, "Final Delay Count In"=w480) -> (w434:T5)
            n29 = Bundle By Name(cluster=w713, "Old Average"=w714, "New Average"=w534, "Current State"=w549, "Detector 1 Correlation"=w643, "Detector 3 Correlation"=w642, "Velocity Count"=w445, "Detector Counter in"=w542, "Timeout Count in"=w646, "Measured Charge in"=w645, "Filter Threshold"="Filter 1 threshold", "High Correlation in"=w644, "Offset"=w531, "Offset Average"=w517, "Measured Velocity In"=w510, "Mult Cluster"=w493, "Delay1 In"=w491, "Final Delay Count In"=w490) -> (w438:T5)
            n30 = Bundle By Name(cluster=w678, "Old Average"=w686, "New Average"=w534, "Current State"=w546, "Detector 1 Correlation"=w628, "Detector 3 Correlation"=w627, "Velocity Count"=w684, "Detector Counter in"=w539, "Timeout Count in"=w681, "Measured Charge in"=w680, "Filter Threshold"="Filter 4 threshold", "High Correlation in"=w631, "Offset"=w522, "Offset Average"=w517, "Measured Velocity In"=w506, "Mult Cluster"=w493, "Delay1 In"=w465, "Final Delay Count In"=w482) -> (w435:T5)
            n31 = Bundle By Name(cluster=w707, "Old Average"=w706, "New Average"=w534, "Current State"=w548, "Detector 1 Correlation"=w638, "Detector 3 Correlation"=w637, "Velocity Count"=w703, "Detector Counter in"=w541, "Timeout Count in"=w702, "Measured Charge in"=w698, "Filter Threshold"="Filter 2 threshold", "High Correlation in"=w639, "Offset"=w526, "Offset Average"=w517, "Measured Velocity In"=w504, "Mult Cluster"=w493, "Delay1 In"=w487, "Final Delay Count In"=w486) -> (w437:T5)
            n32 = Bundle By Name(cluster=w697, "Old Average"=w696, "New Average"=w534, "Current State"=w547, "Detector 1 Correlation"=w633, "Detector 3 Correlation"=w632, "Velocity Count"=w693, "Detector Counter in"=w540, "Timeout Count in"=w691, "Measured Charge in"=w689, "Filter Threshold"="Filter 3 threshold", "High Correlation in"=w634, "Offset"=w525, "Offset Average"=w517, "Measured Velocity In"=w505, "Mult Cluster"=w493, "Delay1 In"=w466, "Final Delay Count In"=w484) -> (w436:T5)
            n33 = Bundle By Name(cluster=T4 {"Separation cut off 1"=4, "Filter Number"=5, "Separation cut off 2"=6} ("Filter Specific Constants"), "Separation cut off 1"=5, "Filter Number"=7, "Separation cut off 2"=0) -> (w448:T4)
            n34 = Bundle By Name(cluster=T4 {"Separation cut off 1"=4, "Filter Number"=5, "Separation cut off 2"=6} ("Filter Specific Constants"), "Separation cut off 1"=0, "Filter Number"=2, "Separation cut off 2"=1) -> (w591:T4)
            n35 = Bundle By Name(cluster=T4 {"Separation cut off 1"=4, "Filter Number"=5, "Separation cut off 2"=6} ("Filter Specific Constants"), "Separation cut off 1"=4, "Filter Number"=6, "Separation cut off 2"=5) -> (w581:T4)
            n36 = Bundle By Name(cluster=T4 {"Separation cut off 1"=4, "Filter Number"=5, "Separation cut off 2"=6} ("Filter Specific Constants"), "Separation cut off 1"=3, "Filter Number"=5, "Separation cut off 2"=4) -> (w583:T4)
            n37 = Bundle By Name(cluster=T4 {"Separation cut off 1"=4, "Filter Number"=5, "Separation cut off 2"=6} ("Filter Specific Constants"), "Separation cut off 1"=0, "Filter Number"=1, "Separation cut off 2"=0) -> (w589:T4)
            n38 = call "filter_logic_delays.vi"("Filter Specific Constants"=w589, "Variables Cluster"=w438, "controls cluster"=w494) -> ("Output Cluster"=w588:T7)  [unwired: 8 in]
            n39 = call "filter_logic_delays.vi"("Filter Specific Constants"=w591, "Variables Cluster"=w437, "controls cluster"=w494) -> ("Output Cluster"=w598:T7)  [unwired: 8 in]
            n40 = Bundle By Name(cluster=T4 {"Separation cut off 1"=4, "Filter Number"=5, "Separation cut off 2"=6} ("Filter Specific Constants"), "Separation cut off 1"=1, "Filter Number"=3, "Separation cut off 2"=2) -> (w587:T4)
            n41 = Bundle By Name(cluster=T4 {"Separation cut off 1"=4, "Filter Number"=5, "Separation cut off 2"=6} ("Filter Specific Constants"), "Separation cut off 1"=2, "Filter Number"=4, "Separation cut off 2"=3) -> (w585:T4)
            n42 = call "filter_logic_delays.vi"("Filter Specific Constants"=w581, "Variables Cluster"=w433, "controls cluster"=w494) -> ("Output Cluster"=w580:T7)  [unwired: 8 in]
            n43 = call "filter_logic_delays.vi"("Filter Specific Constants"=w583, "Variables Cluster"=w434, "controls cluster"=w494) -> ("Output Cluster"=w582:T7)  [unwired: 8 in]
            n44 = call "filter_logic_delays.vi"("Filter Specific Constants"=w587, "Variables Cluster"=w436, "controls cluster"=w494) -> ("Output Cluster"=w586:T7)  [unwired: 8 in]
            n45 = call "filter_logic_delays.vi"("Filter Specific Constants"=w585, "Variables Cluster"=w435, "controls cluster"=w494) -> ("Output Cluster"=w584:T7)  [unwired: 8 in]
            n46 = call "filter_logic_delays.vi"("Filter Specific Constants"=w448, "Variables Cluster"=w432, "controls cluster"=w494) -> ("Output Cluster"=w590:T7)  [unwired: 8 in]
            n47 = Unbundle By Name(w588) -> ("Average Out"=w712:i32, "Next State"=w711:u8, "Velocity Count out"=w612:i32, "Detector counter out"=w710:i32, "Timeout count out"=w709:u32, "Measured Charge Out"=w611:i32, "High Correlation Out"=w708:i32, "Plates"=w556:bool, "Offset Out"=w530:i32, "Measured Velocity Out"=w503:i32, "Delay1"=w474:i32, "Out1"=w468:bool, "Final Delay Count Out"=w492:u16)
            n48 = Unbundle By Name(w598) -> ("Average Out"=w705:i32, "Next State"=w704:u8, "Velocity Count out"=w610:i32, "Detector counter out"=w701:i32, "Timeout count out"=w700:u32, "Measured Charge Out"=w609:i32, "High Correlation Out"=w699:i32, "Plates"=w555:bool, "Offset Out"=w529:i32, "Measured Velocity Out"=w502:i32, "Delay1"=w489:i32, "Out1"=w467:bool, "Final Delay Count Out"=w488:u16)
            n49 = Unbundle By Name(w582) -> ("Average Out"=w676:i32, "Next State"=w674:u8, "Velocity Count out"=w605:i32, "Detector counter out"=w672:i32, "Timeout count out"=w671:u32, "Measured Charge Out"=w604:i32, "High Correlation Out"=w668:i32, "Plates"=w552:bool, "Offset Out"=w521:i32, "Measured Velocity Out"=w499:i32, "Delay1"=w471:i32, "Out1"=w458:bool, "Final Delay Count Out"=w481:u16)
            n50 = Unbundle By Name(w584) -> ("Average Out"=w687:i32, "Next State"=w685:u8, "Velocity Count out"=w535:i32, "Detector counter out"=w683:i32, "Timeout count out"=w682:u32, "Measured Charge Out"=w606:i32, "High Correlation Out"=w679:i32, "Plates"=w553:bool, "Offset Out"=w523:i32, "Measured Velocity Out"=w500:i32, "Delay1"=w472:i32, "Out1"=w459:bool, "Final Delay Count Out"=w483:u16)
            n51 = Unbundle By Name(w590) -> ("Average Out"=w656:i32, "Next State"=w654:u8, "Velocity Count out"=w601:i32, "Detector counter out"=w652:i32, "Timeout count out"=w651:u32, "Measured Charge Out"=w600:i32, "High Correlation Out"=w648:i32, "Plates"=w550:bool, "Offset Out"=w516:i32, "Measured Velocity Out"=w497:i32, "Delay1"=w469:i32, "Out1"=w457:bool, "Final Delay Count Out"=w476:u16)
            n52 = Unbundle By Name(w580) -> ("Average Out"=w666:i32, "Next State"=w665:u8, "Velocity Count out"=w602:i32, "Detector counter out"=w662:i32, "Timeout count out"=w661:u32, "Measured Charge Out"=w603:i32, "High Correlation Out"=w658:i32, "Plates"=w551:bool, "Offset Out"=w519:i32, "Measured Velocity Out"=w498:i32, "Delay1"=w470:i32, "Out1"=w456:bool, "Final Delay Count Out"=w478:u16)
            n53 = Unbundle By Name(w586) -> ("Average Out"=w695:i32, "Next State"=w694:u8, "Velocity Count out"=w608:i32, "Detector counter out"=w692:i32, "Timeout count out"=w690:u32, "Measured Charge Out"=w607:i32, "High Correlation Out"=w688:i32, "Plates"=w554:bool, "Offset Out"=w524:i32, "Measured Velocity Out"=w501:i32, "Delay1"=w473:i32, "Out1"=w460:bool, "Final Delay Count Out"=w485:u16)
            n54 = Select(t=FALSE, s=w428, f="Reset One Shot") -> (s? t:f=w419:bool)
            n55 = Select(t=FALSE, s=w419, f=w410) -> (s? t:f=w431:bool)
            n56 = Not And(1:w431, 2:"One Shot") -> (0:w422:bool)
            n57 = Select(t=FALSE, s=w419, f=w411) -> (s? t:f=w414:bool)
            n58 = Not And(1:w414, 2:"One Shot") -> (0:w420:bool)
            n59 = Compound Arithmetic op=OR(w556, w555, w554, w553, w552, w551, w550) -> (w447:bool)
            n60 = call "delay_sorter.vi"("Out1 1"=w468, "Out1 2"=w467, "Out1 3"=w460, "Out1 4"=w459, "Out1 5"=w458, "Out1 6"=w456, "Out1 7"=w457) -> ("Delay1"=w424:bool)  [unwired: 8 in]
            n61 = Select(t=TRUE, s=w441, f=w422) -> (s? t:f=w439:bool)
            n62 = Select(t=TRUE, s=w417, f=w420) -> (s? t:f=w426:bool)
            n63 = Select(t=w447, s=w439, f=FALSE) -> (s? t:f=w442:bool)
            "Plates" <- w442
            n64 = Select(t=w424, s=w426, f=FALSE) -> (s? t:f=w416:bool)
            "Delay1" <- w416
            n65 = Select(t=TRUE, s=w442, f=w431) -> (s? t:f=w430:bool)
            "Not Armed?" <- w430
            n66 = Select(t=TRUE, s=w416, f=w414) -> (s? t:f=w413:bool)
            "Del Not Armed?" <- w413
          }
        }
      }
      n67 = node-c288(w33) -> ()
      n68 = while {
        stop <- FALSE stop-if-true
        n69 = xnode "FPGA I/O Node"("IO Module\\PFI Enable"=TRUE ("IO Module\\PFI Enable")) -> ()  [unwired: 1 in, 1 out]
        n70 = local read "Plates"() -> (w110:bool)
        n71 = xnode "FPGA I/O Node"("IO Module\\PFI Out 4"=w110) -> ()  [unwired: 1 in, 1 out]
        n72 = local read "Delay1"() -> (w107:bool)
        n73 = xnode "FPGA I/O Node"("IO Module\\PFI Out 1"=w107) -> ()  [unwired: 1 in, 1 out]
      }
      n74 = node-c288(w97) -> ()
    }
  }
